vi "Is Data Modified.vi"(8 "error in (no error)":errorcluster) -> (0 "error out":errorcluster, 3 "Data Modified?":bool)   [LabVIEW 2014, in "Contact Data.lvlib"]
doc: "Returns if there have been changes made to the address book data store since the last save."
uses:
  Contact Data.lvlib
  Command.ctl
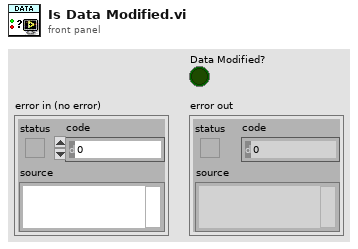
[diagram p1: front panel]
types:
  T1 = typedef "Contact Data.lvlib/Command.ctl" = enum16{"Set All Contacts", "Load", "Save", "Get All Data", "Get Single Data (ID)", "Get Single Data", "Set Position", "Set Destinations", "Set Controls", "Remove Single Data", "Remove UUID Contact", "Set Single ALL", "Is Data Modified", "Import Data"}
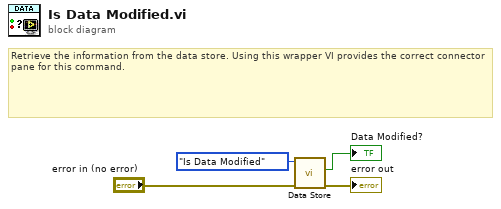
[diagram p0: block diagram]
diagram:
  # "Retrieve the information from the data store. Using this wrapper VI provides the correct connector pane for this command."
  n1 = call "Data Store.vi"("error in (no error)"="error in (no error)", "Command"=Command."Is Data Modified") -> ("error out"=→"error out":errorcluster, "Data Modified?"=→"Data Modified?":bool)  [unwired: 7 in, 1 out]
